vi "Position Waypoint Type Tab.vi"(8 "Error In":errorcluster, 10 "DigNum Refnum":refnum<vi>, 11 "TabCtl Refnum":refnum<vi>) -> (0 "Error Out":errorcluster)   [LabVIEW 2014]
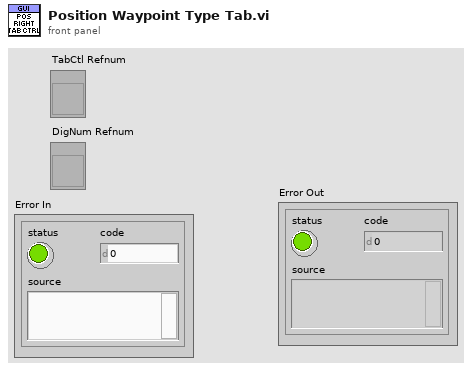
[diagram p1: front panel]
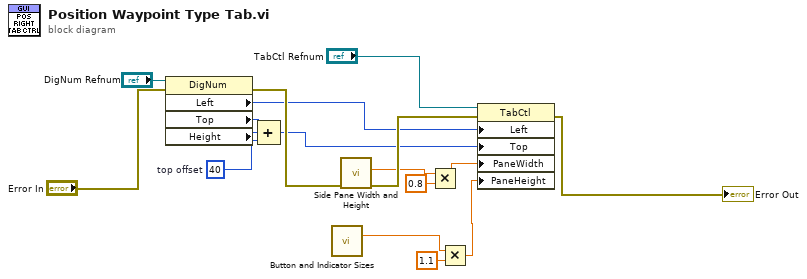
[diagram p0: block diagram]
diagram:
  w4 = u32 40  # top offset
  n1 = property class="DigNum"(reference="DigNum Refnum", error in="Error In") -> (error out=w13:errorcluster, "Left"=w11:i32, "Top"=w10:i32, "Height"=w9:u32)  [unwired: 1 out]
  n2 = Compound Arithmetic op=ADD(w10, w9, w4) -> (w8:u32)
  n3 = call "Button and Indicator Sizes.vi"() -> ("Button Height"=w3:dbl)  [unwired: 11 in, 4 out]
  n4 = call "Side Pane Width and Height.vi"("error in (no error)"=w13) -> ("error out"=w16:errorcluster, "Width"=w7:dbl)  [unwired: 8 in, 1 out]
  n5 = Multiply(x=w7, y=0.8) -> (x*y=w5:dbl)
  n6 = Multiply(x=w3, y=1.1) -> (x*y=w1:dbl)
  n7 = property class="TabCtl"(reference="TabCtl Refnum", error in=w16, "Left"=w11, "Top"=w8, "PaneWidth"=w5, "PaneHeight"=w1) -> (error out=→"Error Out":errorcluster)  [unwired: 1 out]
